vi "DAQmx Analog Trigger Source.vi"(1 "DAQmx Analog Trigger Source":tag) -> (0 "DAQmx Analog Trigger Source Out":tag)   [LabVIEW 2012]
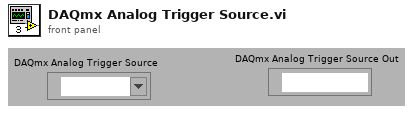
[diagram p1: front panel]
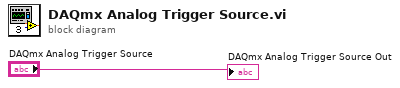
[diagram p0: block diagram]
diagram:
  "DAQmx Analog Trigger Source Out" <- "DAQmx Analog Trigger Source"
